vi "ADS1015_Scale_calculation.vi"(10 "IC Selector":i32(ring)=1 items=["ADS1015"=4096, "AD1115"=65536], 11 "ADS1015 -Gain & Scale":T1(ring)=enum."FS=+/-4.096 V") -> (3 "Scale Value (mV)":dbl)   [LabVIEW 2018]
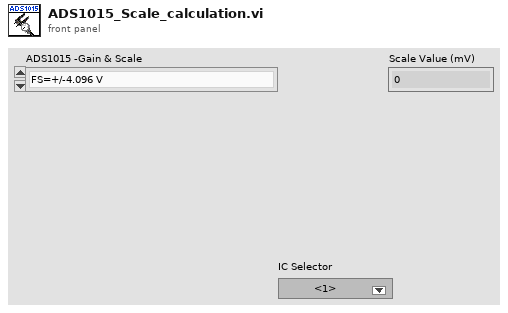
[diagram p1: front panel]
types:
  T1 = enum8{"FS=+/-6.144 V", "FS=+/-4.096 V", "FS=+/-2.048 V", "FS=+/-1.024 V", "FS=+/-0.512 V", "FS=+/-0.256-A V", "FS=+/-0.256-B V", "FS=+/-0.256-C V"}
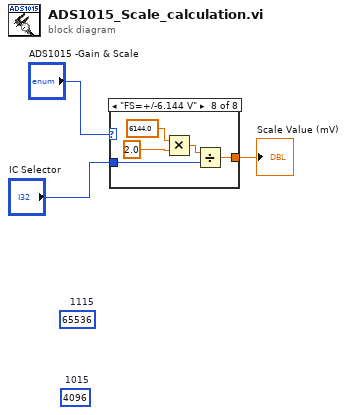
[diagram p0: block diagram]
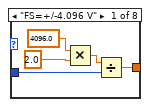
[diagram p2: hidden frame]
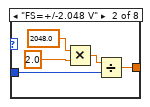
[diagram p3: hidden frame]
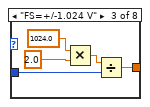
[diagram p4: hidden frame]
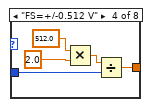
[diagram p5: hidden frame]
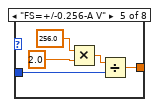
[diagram p6: hidden frame]
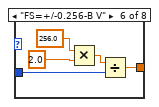
[diagram p7: hidden frame]
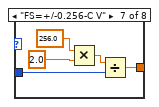
[diagram p8: hidden frame]
diagram:
  (unwired) 4096  # 1015
  (unwired) 65536  # 1115
  n1 = case shown="\"FS=+/-6.144 V\"" "ADS1015 -Gain & Scale" {
    tunnel: "IC Selector" -> [w8 w13 w18 w23 w28 w33 w38 w43]
    tunnel: [w4 w9 w14 w19 w24 w29 w34 w39] -> w3
    frame "FS=+/-4.096 V" {
      n2 = Multiply(x=4096.0, y=2.0) -> (x*y=w5:dbl)
      n3 = Divide(x=w5, y=w8) -> (x/y=w4:dbl)
    }
    frame "FS=+/-2.048 V" {
      n4 = Multiply(x=2048.0, y=2.0) -> (x*y=w10:dbl)
      n5 = Divide(x=w10, y=w13) -> (x/y=w9:dbl)
    }
    frame "FS=+/-1.024 V" {
      n6 = Multiply(x=1024.0, y=2.0) -> (x*y=w15:dbl)
      n7 = Divide(x=w15, y=w18) -> (x/y=w14:dbl)
    }
    frame "FS=+/-0.512 V" {
      n8 = Multiply(x=512.0, y=2.0) -> (x*y=w20:dbl)
      n9 = Divide(x=w20, y=w23) -> (x/y=w19:dbl)
    }
    frame "FS=+/-0.256-A V" {
      n10 = Multiply(x=256.0, y=2.0) -> (x*y=w25:dbl)
      n11 = Divide(x=w25, y=w28) -> (x/y=w24:dbl)
    }
    frame "FS=+/-0.256-B V" {
      n12 = Multiply(x=256.0, y=2.0) -> (x*y=w30:dbl)
      n13 = Divide(x=w30, y=w33) -> (x/y=w29:dbl)
    }
    frame "FS=+/-0.256-C V" {
      n14 = Multiply(x=256.0, y=2.0) -> (x*y=w35:dbl)
      n15 = Divide(x=w35, y=w38) -> (x/y=w34:dbl)
    }
    frame "FS=+/-6.144 V" {
      n16 = Multiply(x=6144.0, y=2.0) -> (x*y=w40:dbl)
      n17 = Divide(x=w40, y=w43) -> (x/y=w39:dbl)
    }
  }
  "Scale Value (mV)" <- w3
